vi "MeasAction.vi"(8 "Errin (no error)":errorcluster caption="entrée d'erreur (pas d'erreur)", 9 "CurvePointIndex":i32, 10 "AllPointIndex":i32, 11 "DefaultDevIn":refnum<class "SR830.lvclass"> caption="DNL_LabVIEW Object in") -> (0 "error out":errorcluster caption="sortie d'erreur", 2 "MeasDatOut":dbl[](array[numeric]), 3 "DefaultDevOut":refnum<class "SR830.lvclass"> caption="DNL_LabVIEW Object out")   [LabVIEW 2012, in "SR830.lvclass"]
uses:
  SR830.lvclass
  SR830.lvclass/SR830.ctl
  BaseDevice/Accessor/GetClassEvent.vi
  BaseDevice/Accessor/GetClassQueue.vi
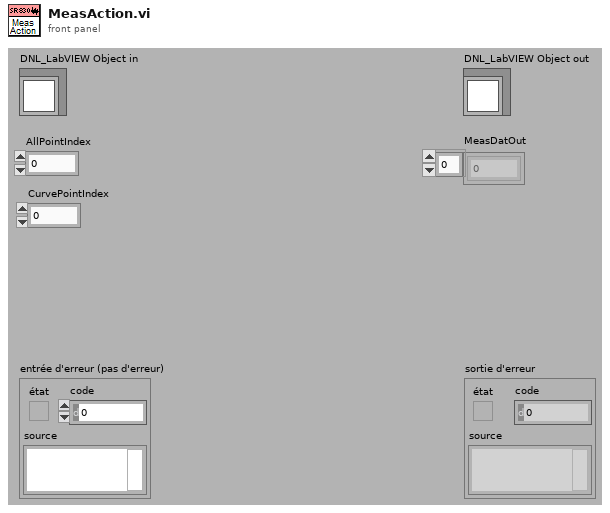
[diagram p1: front panel]
types:
  T1 = typedef "SR830.lvclass/SR830_Func.ctl" = enum16{"Read X & Y (V,V)", "Read Mag & Phase (V,°)", "Read X,Y,Mag & Phase (V,V,V,°)", "Read THz Pump Off/On (V,V,V,°,V,V,V,°,V)"}
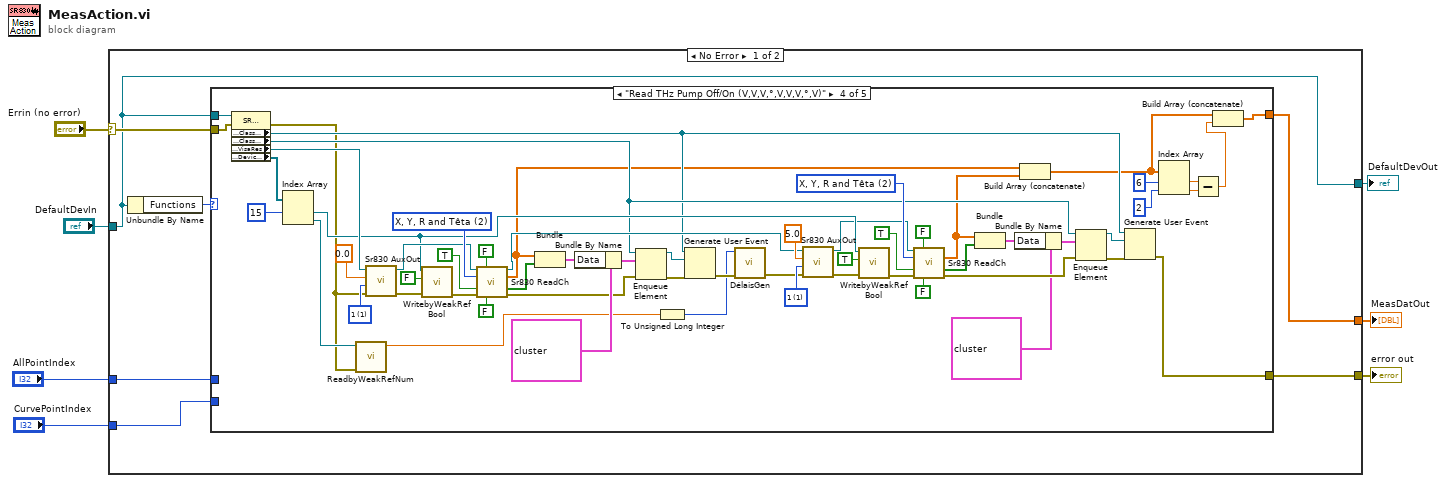
[diagram p0: block diagram]
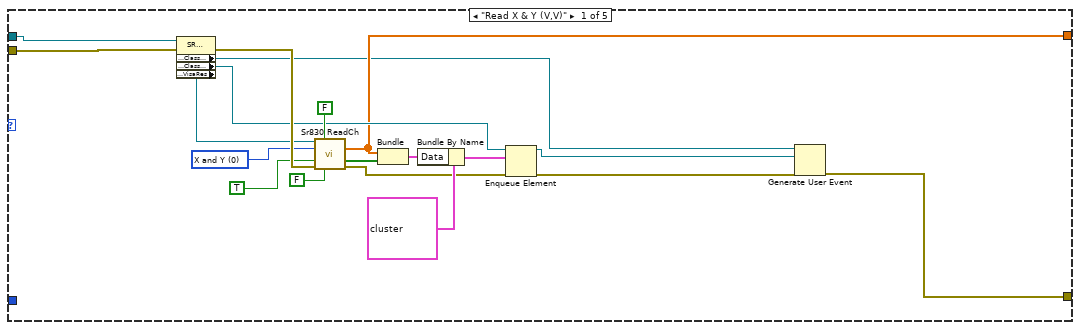
[diagram p2: hidden frame]
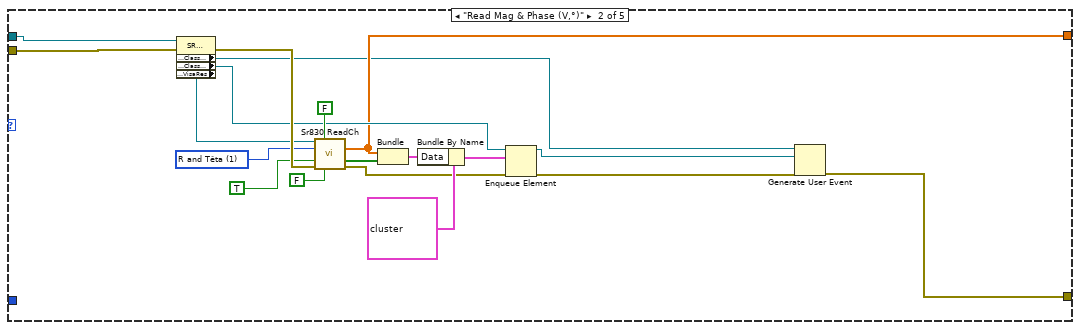
[diagram p3: hidden frame]
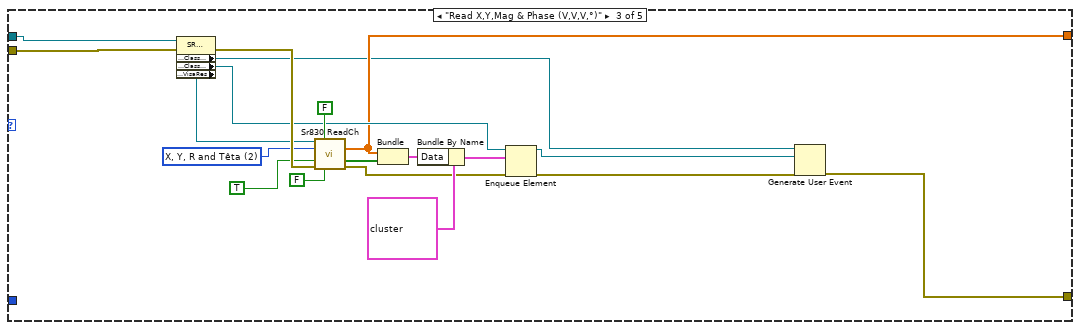
[diagram p4: hidden frame]
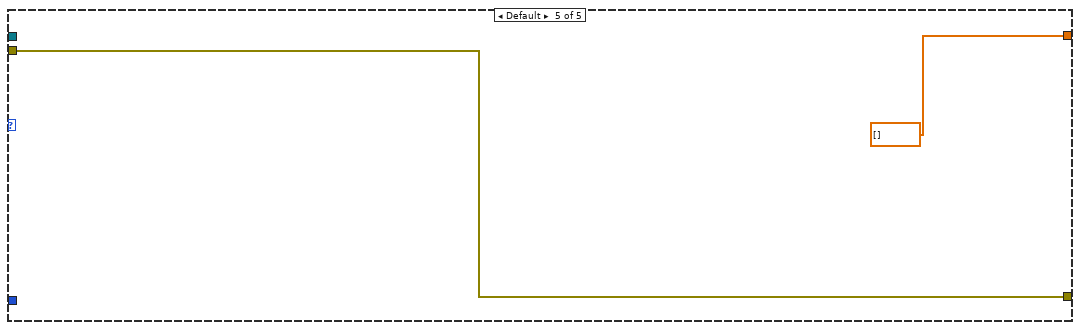
[diagram p5: hidden frame]
diagram:
  n1 = case shown="No Error" "Errin (no error)" {
    selector: "Errin (no error)" -> [w10 w133]
    tunnel: "DefaultDevIn" -> [w8 w134]
    tunnel: [w8 w134] -> w5
    tunnel: "AllPointIndex" -> [w14 _]
    tunnel: [w13 w133] -> w3
    tunnel: [w12 _] -> w2
    tunnel: "CurvePointIndex" -> [w9 _]
    frame No Error {
      n2 = Unbundle By Name(w8) -> ("Functions"=w11:T1)
      n3 = case shown="\"Read THz Pump Off/On (V,V,V,°,V,V,V,°,V)\"" w11 {
        tunnel: w14 -> [_ _ _ _ _]
        tunnel: [w16 w35 w54 w88 w131] -> w13
        tunnel: [w23 w42 w61 w75 dbl[] [] ("Outputs")] -> w12
        tunnel: w10 -> [w32 w51 w70 w129 w131]
        tunnel: w9 -> [_ _ _ _ _]
        tunnel: w8 -> [w33 w52 w71 w130 _]
        frame "Read X & Y (V,V)" {
          w30 = u16 0 items=["X and Y", "R and Têta", "X, Y, R and Têta"] ("Channels")
          n4 = property class="SR830.lvclass"(reference=w33, error in=w32) -> (error out=w31:errorcluster, "Accessor:ClassEvent"=w19:refnum<user-event>, "Accessor:ClassQueue"=w26:refnum<queue>, "Accessor:VisaRes"=w15:refnum<visa-resource-name>)  [unwired: 1 out]
          n5 = call <userlib>:"Sr830 ReadCh.vi"("VISA Rsrc"=w15, "Autoscale"=FALSE, "Channels"=w30, "Check Status"=TRUE, "error in (no error)"=w31, "Ask Correction"=FALSE) -> ("Outputs"=w23:dbl[], "Status Byte"=w22:bool[], "error out"=w20:errorcluster)  [unwired: 4 in, 3 out]
          n6 = Bundle("Outputs"=w23, "Status Byte"=w22) -> (w21:cluster{"Outputs":dbl[], "Status Byte":bool[]})  [unwired: 1 in]
          n7 = Bundle By Name(cluster=cluster{"Message":string, "Data":variant, i32} {"Message"="MeasDone", "Data"=variant, 0} ("élément"), "Data"=w21) -> (w24:cluster{"Message":string, "Data":variant, i32})
          n8 = Enqueue Element(queue=w26, element=w24, error in (no error)=w20) -> (queue out=w17:refnum<queue>, error out=w18:errorcluster)  [unwired: 1 in, 1 out]
          n9 = Generate User Event(user event=w19, event data cluster=w17, error in=w18) -> (error out=w16:errorcluster)  [unwired: 1 out]
        }
        frame "Read Mag & Phase (V,°)" {
          w49 = u16 1 items=["X and Y", "R and Têta", "X, Y, R and Têta"] ("Channels")
          n10 = property class="SR830.lvclass"(reference=w52, error in=w51) -> (error out=w50:errorcluster, "Accessor:ClassEvent"=w38:refnum<user-event>, "Accessor:ClassQueue"=w45:refnum<queue>, "Accessor:VisaRes"=w34:refnum<visa-resource-name>)  [unwired: 1 out]
          n11 = call <userlib>:"Sr830 ReadCh.vi"("VISA Rsrc"=w34, "Autoscale"=FALSE, "Channels"=w49, "Check Status"=TRUE, "error in (no error)"=w50, "Ask Correction"=FALSE) -> ("Outputs"=w42:dbl[], "Status Byte"=w41:bool[], "error out"=w39:errorcluster)  [unwired: 4 in, 3 out]
          n12 = Bundle("Outputs"=w42, "Status Byte"=w41) -> (w40:cluster{"Outputs":dbl[], "Status Byte":bool[]})  [unwired: 1 in]
          n13 = Bundle By Name(cluster=cluster{"Message":string, "Data":variant, i32} {"Message"="MeasDone", "Data"=variant, 0} ("élément"), "Data"=w40) -> (w43:cluster{"Message":string, "Data":variant, i32})
          n14 = Enqueue Element(queue=w45, element=w43, error in (no error)=w39) -> (queue out=w36:refnum<queue>, error out=w37:errorcluster)  [unwired: 1 in, 1 out]
          n15 = Generate User Event(user event=w38, event data cluster=w36, error in=w37) -> (error out=w35:errorcluster)  [unwired: 1 out]
        }
        frame "Read X,Y,Mag & Phase (V,V,V,°)" {
          w68 = u16 2 items=["X and Y", "R and Têta", "X, Y, R and Têta"] ("Channels")
          n16 = property class="SR830.lvclass"(reference=w71, error in=w70) -> (error out=w69:errorcluster, "Accessor:ClassEvent"=w57:refnum<user-event>, "Accessor:ClassQueue"=w64:refnum<queue>, "Accessor:VisaRes"=w53:refnum<visa-resource-name>)  [unwired: 1 out]
          n17 = call <userlib>:"Sr830 ReadCh.vi"("VISA Rsrc"=w53, "Autoscale"=FALSE, "Channels"=w68, "Check Status"=TRUE, "error in (no error)"=w69, "Ask Correction"=FALSE) -> ("Outputs"=w61:dbl[], "Status Byte"=w60:bool[], "error out"=w58:errorcluster)  [unwired: 4 in, 3 out]
          n18 = Bundle("Outputs"=w61, "Status Byte"=w60) -> (w59:cluster{"Outputs":dbl[], "Status Byte":bool[]})  [unwired: 1 in]
          n19 = Bundle By Name(cluster=cluster{"Message":string, "Data":variant, i32} {"Message"="MeasDone", "Data"=variant, 0} ("élément"), "Data"=w59) -> (w62:cluster{"Message":string, "Data":variant, i32})
          n20 = Enqueue Element(queue=w64, element=w62, error in (no error)=w58) -> (queue out=w55:refnum<queue>, error out=w56:errorcluster)  [unwired: 1 in, 1 out]
          n21 = Generate User Event(user event=w57, event data cluster=w55, error in=w56) -> (error out=w54:errorcluster)  [unwired: 1 out]
        }
        frame "Read THz Pump Off/On (V,V,V,°,V,V,V,°,V)" {
          w105 = u16 1 items=["1"=1, "2"=2, "3"=3, "4"=4] ("AuxOut Ch")
          w94 = u16 2 items=["X and Y", "R and Têta", "X, Y, R and Têta"] ("Channels")
          w116 = u16 1 items=["1"=1, "2"=2, "3"=3, "4"=4] ("AuxOut Ch")
          w128 = u16 2 items=["X and Y", "R and Têta", "X, Y, R and Têta"] ("Channels")
          n22 = property class="SR830.lvclass"(reference=w130, error in=w129) -> (error out=w77:errorcluster, "Accessor:ClassEvent"=w89:refnum<user-event>, "Accessor:ClassQueue"=w90:refnum<queue>, "Accessor:VisaRes"=w117:refnum<visa-resource-name>, "Accessor:DeviceCtrl"=w114:refnum<vi>[])  [unwired: 1 out]
          n23 = Index Array(array=w114, index #1=15 ("index")) -> (element #1=w91:refnum<vi>, element #2=w78:refnum<vi>)  [unwired: 1 in]
          n24 = call <userlib>:"ReadbyWeakRefNum.vi"("error in"=w77, "Control Ref"=w78) -> ("Valeur"=w76:dbl)  [unwired: 8 in, 1 out]
          n25 = call <userlib>:"Sr830 AuxOut.vi"("error in"=w77, "AuxOut Ch"=w116, "Voltage"=0.0, "Ressource VISA"=w117) -> ("error out"=w112:errorcluster, "Ressource VISA Out"=w93:refnum<visa-resource-name>)  [unwired: 1 in, 1 out]
          n26 = call <userlib>:"WritebyWeakRefBool.vi"("error in"=w112, "Valeur"=FALSE, "Control Ref"=w91) -> ("error out"=w111:errorcluster)  [unwired: 8 in]
          n27 = call <userlib>:"Sr830 ReadCh.vi"("VISA Rsrc"=w93, "Autoscale"=FALSE, "Channels"=w128, "Check Status"=TRUE, "error in (no error)"=w111, "Ask Correction"=FALSE) -> ("Ressource VISA Out"=w92:refnum<visa-resource-name>, "Outputs"=w85:dbl[], "Status Byte"=w122:bool[], "error out"=w120:errorcluster)  [unwired: 4 in, 2 out]
          n28 = Bundle("Outputs"=w85, "Status Byte"=w122) -> (w121:cluster{"Outputs":dbl[], "Status Byte":bool[]})  [unwired: 1 in]
          n29 = Bundle By Name(cluster=cluster{"Message":string, "Data":variant, i32} {"Message"="MeasDone", "Data"=variant, 0} ("élément"), "Data"=w121) -> (w123:cluster{"Message":string, "Data":variant, i32})
          n30 = Enqueue Element(queue=w90, element=w123, error in (no error)=w120) -> (queue out=w118:refnum<queue>, error out=w119:errorcluster)  [unwired: 1 in, 1 out]
          n31 = To Unsigned Long Integer(number=w76) -> (unsigned 32bit integer=w73:u32)
          n32 = Generate User Event(user event=w89, event data cluster=w118, error in=w119) -> (error out=w87:errorcluster)  [unwired: 1 out]
          n33 = call "DélaisGen.vi"("error in (no error)"=w87, "ms To Wait"=w73) -> ("error out"=w86:errorcluster)  [unwired: 9 in]
          n34 = call <userlib>:"Sr830 AuxOut.vi"("error in"=w86, "AuxOut Ch"=w105, "Voltage"=5.0, "Ressource VISA"=w92) -> ("error out"=w107:errorcluster, "Ressource VISA Out"=w72:refnum<visa-resource-name>)  [unwired: 1 in, 1 out]
          n35 = call <userlib>:"WritebyWeakRefBool.vi"("error in"=w107, "Valeur"=TRUE, "Control Ref"=w91) -> ("error out"=w108:errorcluster)  [unwired: 8 in]
          n36 = call <userlib>:"Sr830 ReadCh.vi"("VISA Rsrc"=w72, "Autoscale"=FALSE, "Channels"=w94, "Check Status"=TRUE, "error in (no error)"=w108, "Ask Correction"=FALSE) -> ("Outputs"=w79:dbl[], "Status Byte"=w100:bool[], "error out"=w102:errorcluster)  [unwired: 4 in, 3 out]
          n37 = Bundle("Outputs"=w79, "Status Byte"=w100) -> (w101:cluster{"Outputs":dbl[], "Status Byte":bool[]})  [unwired: 1 in]
          n38 = Bundle By Name(cluster=cluster{"Message":string, "Data":variant, i32} {"Message"="MeasDone", "Data"=variant, 0} ("élément"), "Data"=w101) -> (w99:cluster{"Message":string, "Data":variant, i32})
          n39 = Build Array (concatenate)(w85, w79) -> (w80:dbl[])
          n40 = Enqueue Element(queue=w90, element=w99, error in (no error)=w102) -> (queue out=w104:refnum<queue>, error out=w103:errorcluster)  [unwired: 1 in, 1 out]
          n41 = Generate User Event(user event=w89, event data cluster=w104, error in=w103) -> (error out=w88:errorcluster)  [unwired: 1 out]
          n42 = Index Array(array=w80, index #1=6 ("index"), index #2=2 ("index")) -> (element #1=w81:dbl, element #2=w82:dbl)
          n43 = Subtract(x=w81, y=w82) -> (x-y=w74:dbl)
          n44 = Build Array (concatenate)(w80, w74) -> (w75:dbl[])
        }
        frame Default {
        }
      }
    }
    frame Error {
    }
  }
  "error out" <- w3
  "DefaultDevOut" <- w5
  "MeasDatOut" <- w2
